vi "co-pilot set motor power.vi"(11 "MechanismMetrics":T1) -> (0 "MechanismMetrics 2":T1, 8 "Waveform Chart":dbl(graph))   [LabVIEW 2014]
uses:
  MechanismMetrics.ctl
  Lifter States.ctl
  Auto Lifter States.ctl
  limitSwitchGlobals.vi
panel:
  in  "Power":dbl
  in  "Calibrate":bool
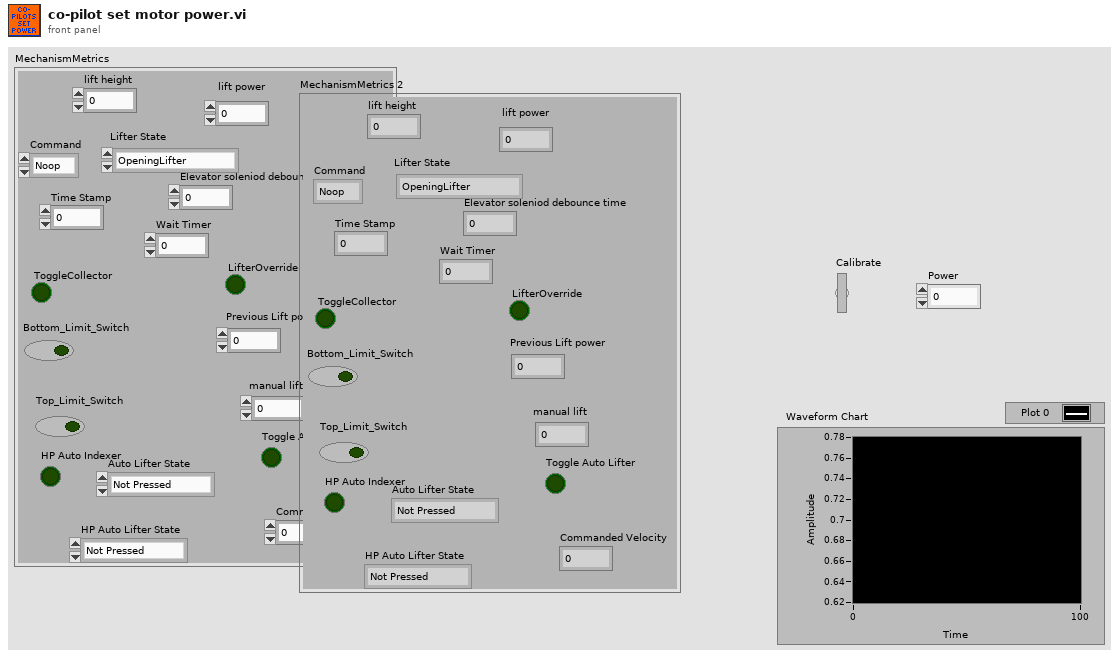
[diagram p1: front panel]
types:
  T1 = typedef "MechanismMetrics.ctl" = cluster{"lift height":dbl, "Command":enum16{"Noop", "Flagged"}, "Time Stamp":u32, "ToggleCollector":bool, "Bottom_Limit_Switch ":bool, "Top_Limit_Switch":bool, "lift power":dbl, "Elevator soleniod debounce time   ":dbl, "LifterOverride":bool, "Previous Lift power":dbl, "manual lift":dbl, "Lifter State":T2, "Auto Lifter State":T3, "Toggle Auto Lifter":bool, "Wait Timer":dbl, "HP Auto Indexer":bool, "HP Auto Lifter State":T3, "Commanded Velocity":dbl}
  T2 = typedef "Lifter States.ctl" = enum16{"OpeningLifter", "LifterOpen", "ClosingLifter", "LifterClosed"}
  T3 = typedef "Auto Lifter States.ctl" = enum16{"Not Pressed", "THE_END", "WAIT_FOR_RELEASE", "Press Detected", "To Release Stacked1", "To Collect", "Open Lifter", "WAIT", "Close", "To Stack1"}
  T4 = typedef "WPI_MotorControlDeviceRef.ctl" = cluster{"DeviceStatus":errorcluster, "Type":T5, "PWM":cluster{"Controller":T6, "PWM Channel":T7, "DeadBand":T8}, "CAN":cluster{"Device Number":u8, "Control Mode":T9, "Semaphore":T10, "Max Vout":dbl, "TalonSRX Control Mode":T11}, "Invert":bool, "TransformRef":T12, "InvTransformRef":T12}
  T5 = typedef "WPI_MotorControlType.ctl" = enum16{"PWM", "CAN", "CANTalonSRX"}
  T6 = typedef "FPGA_TypedefDigitalModule.ctl" = enum16{"Controller 1"}
  T7 = typedef "FPGA_DIOPWMChannel.ctl" = enum8{"PWM 0", "PWM 1", "PWM 2", "PWM 3", "PWM 4", "PWM 5", "PWM 6", "PWM 7", "PWM 8", "PWM 9", "PWM MXP 0", "PWM MXP 1", "PWM MXP 2", "PWM MXP 3", "PWM MXP 4", "PWM MXP 5", "PWM MXP 6", "PWM MXP 7", "PWM MXP 8", "PWM MXP 9", "Invalid"}
  T8 = typedef "WPI_PWMDeadband.ctl" = cluster{"Name":string, "maxPositivePwm":i32, "minPositivePwm":i32, "centerPwm":i32, "maxNegativePwm":i32, "minNegativePwm":i32, "angularRange":u16}
  T9 = typedef "WPI_CANJaguar_ControlMode.ctl" = enum8{"Percent VBus", "Current", "Speed", "Position", "Voltage"}
  T10 = typedef "Semaphore RefNum" = refnum<k1>
  T11 = typedef "WPI_CANTalonSRX_APIControlMode.ctl" = enum8{"Percent VBus", "Speed", "Position", "Slave", "Unchanged / Invalid"}
  T12 = typedef "WPI_PWMTransform_ConPane.ctl" = refnum<vi>
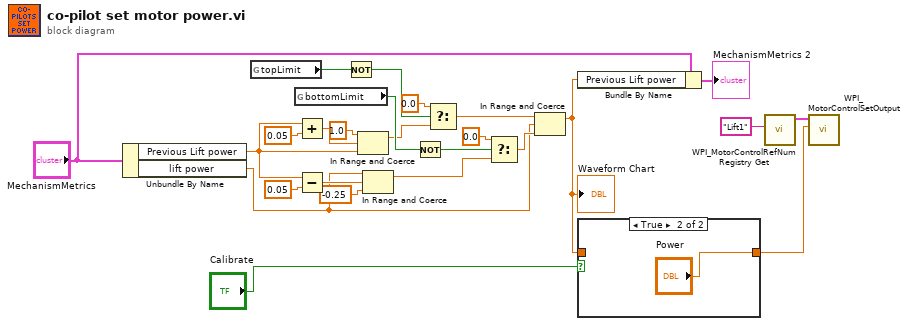
[diagram p0: block diagram]
diagram:
  n1 = Unbundle By Name("MechanismMetrics") -> ("Previous Lift power"=w3:dbl, "lift power"=w2:dbl)
  n2 = global read "limitSwitchGlobals.vi" "topLimit"() -> (w17:bool)
  n3 = global read "limitSwitchGlobals.vi" "bottomLimit"() -> (w18:bool)
  n4 = Add(x=w3, y=0.05) -> (x+y=w10:dbl)
  n5 = Subtract(x=w3, y=0.05) -> (x-y=w13:dbl)
  n6 = Not(x=w17) -> (.not. x?=w6:bool)
  n7 = In Range and Coerce(upper limit=1.0, x=w10, lower limit=w3) -> (coerced(x)=w9:dbl)  [unwired: 1 out]
  n8 = In Range and Coerce(upper limit=w2, x=w13, lower limit=-0.25 ("f")) -> (coerced(x)=w12:dbl)  [unwired: 1 out]
  n9 = Not(x=w18) -> (.not. x?=w7:bool)
  n10 = Select(t=0.0, s=w6, f=w9) -> (s? t:f=w21:dbl)
  n11 = Select(t=0.0, s=w7, f=w12) -> (s? t:f=w19:dbl)
  n12 = In Range and Coerce(upper limit=w21, x=w2, lower limit=w19) -> (coerced(x)=w5:dbl)  [unwired: 1 out]
  "Waveform Chart" <- w5
  n13 = Bundle By Name(cluster="MechanismMetrics", "Previous Lift power"=w5) -> (→"MechanismMetrics 2":T1)
  n14 = case shown="True" "Calibrate" {
    tunnel: w5 -> [w26 _]
    tunnel: [w26 "Power"] -> w4
    frame False {
    }
    frame True {
    }
  }
  n15 = call <vilib>:"WPI_MotorControlRefNum Registry Get.vi"("refnum name"="Lift1") -> ("MotorControlDevRef"=w25:T4)  [unwired: 9 in, 1 out]
  n16 = call <vilib>:"WPI_MotorControlSetOutput.vi"("Output"=w4, "MotorControlDevRef"=w25) -> ()  [unwired: 7 in, 3 out]
